vi "populate kvp table.vi"(8 "error in":errorcluster, 11 "fixed channel configuration in":refnum<class "control module configuration.lvclass">) -> (0 "error out":errorcluster, 2 "kvp's":string[][](array[string]), 3 "fixed channel configuration out":refnum<class "control module configuration.lvclass">)   [LabVIEW 2013, in "control module editor.lvclass"]
uses:
  control module editor.lvclass
  configuration/control module configuration.lvclass
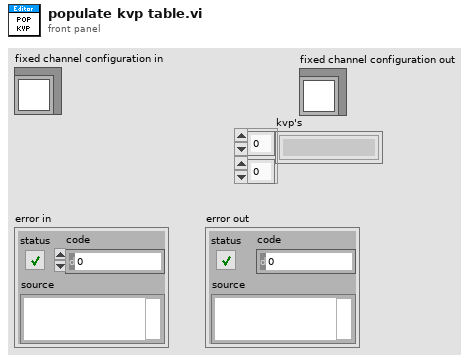
[diagram p1: front panel]
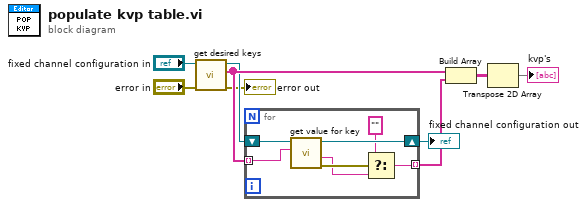
[diagram p0: block diagram]
diagram:
  n1 = call-dynamic "get desired keys.vi"("error in"="error in", "fixed channel configuration in"="fixed channel configuration in") -> ("error out"=→"error out":errorcluster, "desired keys"=w9:string[], "fixed channel configuration out"=w6:refnum<class "control module configuration.lvclass">)  [unwired: 7 in]
  n2 = for {
    shift-right: [w15] -> w1
    shift-left: w6 -> [w16]
    tunnel: w9 -> [w14] mode=indexing
    tunnel: [w11] -> w7 mode=indexing
    n3 = call-dynamic "get value for key.vi"("key"=w14, "fixed channel configuration in"=w16) -> ("error out"=w13:errorcluster, "value"=w12:string, "fixed channel configuration out"=w15:refnum<class "control module configuration.lvclass">)  [unwired: 7 in]
    n4 = Select(t="", s=w13, f=w12) -> (s? t:f=w11:string)
  }
  "fixed channel configuration out" <- w1
  n5 = Build Array(w9, w7) -> (w8:string[][])
  n6 = Transpose 2D Array(2D array=w8) -> (transposed array=→"kvp's":string[][])
